vi "AssertsGreater.vi"(0 "VI Reference In":refnum<vi>, 1 "Label (VI Title)":string="Default", 11 "error in (no error)":errorcluster) -> (4 "VI Reference Out":refnum<vi>, 15 "error out":errorcluster)   [LabVIEW 2016, in "DronaTest.lvlib"]
uses:
  DronaTest.lvlib
  main/apis/Stimulus/KeyBoardSimulation/ValueSignalLatchBooleanString.vi
  main/apis/Assert/AssertControlValue/Greater.vi
  <vilib>/addons/_JKI Toolkits/Caraya/classes/Assert/Assert Error.vi
  <vilib>/addons/_JKI Toolkits/Caraya/classes/Assert/Assert Not Error.vi
  main/apis/Assert/AssertControlValue/GreaterOrEqual.vi
  <vilib>/addons/_JKI Toolkits/Caraya/classes/Test/Test.lvclass
  main/Drona.lvlib
  <vilib>/addons/_JKI Toolkits/Caraya/classes/Assert/Assert.lvclass
  main/apis/Stimulus/KeyBoardSimulation/KeyboardSimulation.lvlib
  main/apis/Assert/AssertControlValue/AssertControlValue.lvlib
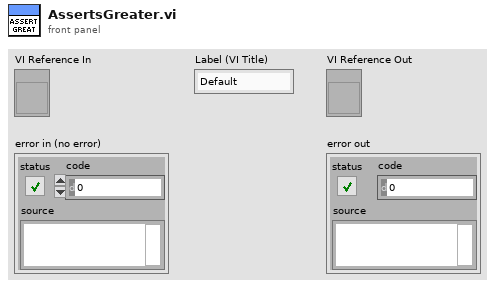
[diagram p1: front panel]
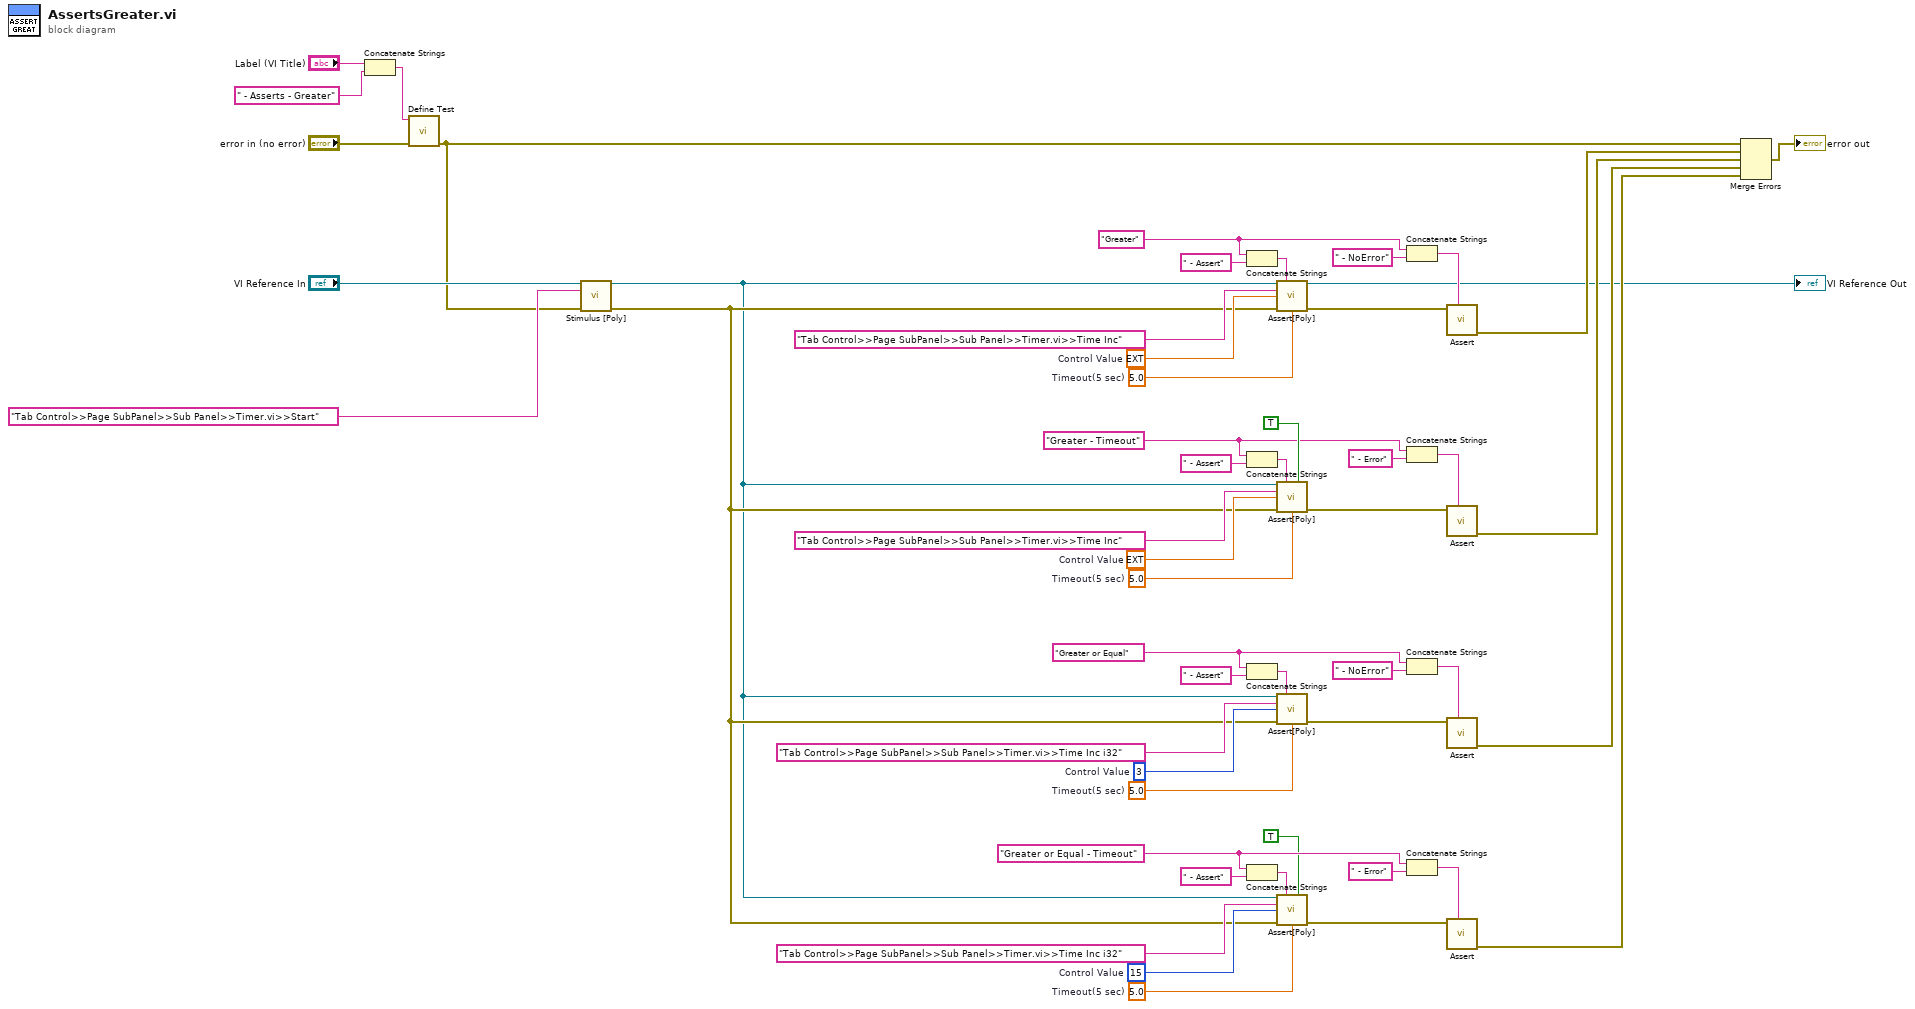
[diagram p0: block diagram]
diagram:
  w16 = 5.0  # Timeout(5 sec)
  w17 = 3  # Control Value
  w18 = "Greater or Equal" ("string")
  w15 = 5.0  # Timeout(5 sec)
  w14 = 15  # Control Value
  w13 = "Greater or Equal - Timeout" ("string")
  w33 = 5.0  # Timeout(5 sec)
  w32 = ext 3.0  # Control Value
  w31 = "Greater" ("string")
  w34 = 5.0  # Timeout(5 sec)
  w35 = ext 15.0  # Control Value
  w36 = "Greater - Timeout" ("string")
  n1 = Concatenate Strings("Label (VI Title)", " - Asserts - Greater" ("Label (VI Title)")) -> (w49:string)
  n2 = call <vilib>:"Define Test.vi"("error in (no error)"="error in (no error)", "Label (VI Title)"=w49) -> ("error out"=w46:errorcluster)  [unwired: 9 in]
  n3 = call-poly "Stimulus [Poly].vi"("VI Reference In"="VI Reference In", "Control Path"="Tab Control>>Page SubPanel>>Sub Panel>>Timer.vi>>Start", "error in"=w46) -> ("VI Reference Out"=w2:refnum<vi>, "error out"=w3:errorcluster)  [unwired: 11 in]
  n4 = Concatenate Strings(w31, " - Assert" ("string")) -> (w29:string)
  n5 = Concatenate Strings(w36, " - Assert" ("string")) -> (w38:string)
  n6 = Concatenate Strings(w18, " - Assert" ("string")) -> (w20:string)
  n7 = Concatenate Strings(w13, " - Assert" ("string")) -> (w11:string)
  n8 = call-poly "Assert[Poly].vi"("VI Reference In"=w2, "Label"=w29, "Control Path"="Tab Control>>Page SubPanel>>Sub Panel>>Timer.vi>>Time Inc", "Control Value"=w32, "Error In"=w3, "Timeout(5 sec)"=w33) -> ("VI Reference Out"=→"VI Reference Out":refnum<vi>, "Error Out"=w28:errorcluster)  [unwired: 8 in]
  n9 = call-poly "Assert[Poly].vi"("VI Reference In"=w2, "Label"=w38, "Assert Only? (F)"=TRUE, "Control Path"="Tab Control>>Page SubPanel>>Sub Panel>>Timer.vi>>Time Inc", "Control Value"=w35, "Error In"=w3, "Timeout(5 sec)"=w34) -> ("Error Out"=w39:errorcluster)  [unwired: 7 in, 1 out]
  n10 = call-poly "Assert[Poly].vi"("VI Reference In"=w2, "Label"=w20, "Control Path"="Tab Control>>Page SubPanel>>Sub Panel>>Timer.vi>>Time Inc i32", "Control Value"=w17, "Error In"=w3, "Timeout(5 sec)"=w16) -> ("Error Out"=w21:errorcluster)  [unwired: 8 in, 1 out]
  n11 = call-poly "Assert[Poly].vi"("VI Reference In"=w2, "Label"=w11, "Assert Only? (F)"=TRUE, "Control Path"="Tab Control>>Page SubPanel>>Sub Panel>>Timer.vi>>Time Inc i32", "Control Value"=w14, "Error In"=w3, "Timeout(5 sec)"=w15) -> ("Error Out"=w10:errorcluster)  [unwired: 7 in, 1 out]
  n12 = Concatenate Strings(w31, " - NoError" ("string")) -> (w30:string)
  n13 = Concatenate Strings(w36, " - Error" ("string")) -> (w37:string)
  n14 = Concatenate Strings(w18, " - NoError" ("string")) -> (w19:string)
  n15 = Concatenate Strings(w13, " - Error" ("string")) -> (w12:string)
  n16 = call-poly <vilib>:"Assert.vi"("Label"=w30, "Not Error?"=w28) -> ("error out"=w45:errorcluster)  [unwired: 9 in]
  n17 = call-poly <vilib>:"Assert.vi"("Label"=w37, "Error?"=w39) -> ("error out"=w44:errorcluster)  [unwired: 9 in]
  n18 = call-poly <vilib>:"Assert.vi"("Label"=w19, "Not Error?"=w21) -> ("error out"=w5:errorcluster)  [unwired: 9 in]
  n19 = call-poly <vilib>:"Assert.vi"("Label"=w12, "Error?"=w10) -> ("error out"=w4:errorcluster)  [unwired: 9 in]
  n20 = Merge Errors(w46, w45, w44, w5, w4) -> (→"error out":errorcluster)
